vi "Read_Temp_Omega.vi"(11 "VISA Omega (Serial - COM1)":refnum<visa-resource-name>) -> (0 "error out":errorcluster, 3 "Temperature":dbl)   [LabVIEW 2012]
uses:
  <vilib>/Instr/_visa.llb/VISA Configure Serial Port (Instr).vi
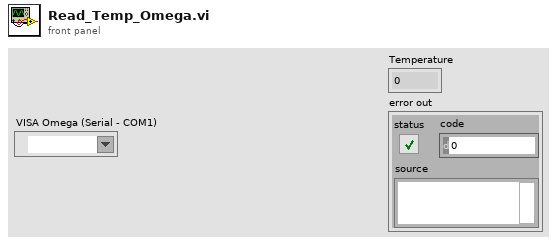
[diagram p1: front panel]
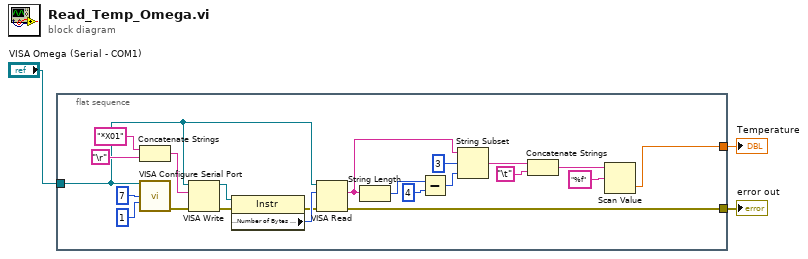
[diagram p0: block diagram]
diagram:
  n1 = flat-sequence {
    tunnel: "VISA Omega (Serial - COM1)" -> [w6]
    tunnel: [w5] -> w1
    tunnel: [w4] -> w2
    frame #0 {
      n2 = Concatenate Strings("*X01", "\r") -> (w14:string)
      n3 = call-poly "VISA Configure Serial Port"("VISA resource name"=w6, "data bits (8)"=7, "parity (0:none)"=1) -> ("error out"=w11:errorcluster)  [unwired: 11 in, 1 out]
      n4 = VISA Write(VISA resource name=w6, write buffer=w14, error in (no error)=w11) -> (VISA resource name out=w25:refnum<visa-resource-name>, error out=w15:errorcluster)  [unwired: 1 out]
      n5 = property class="Instr"(reference=w25, error in=w15) -> (error out=w16:errorcluster, "Serial Settings:Number of Bytes at Serial Port"=w17:u32)  [unwired: 1 out]
      n6 = VISA Read(VISA resource name=w6, byte count=w17, error in (no error)=w16) -> (read buffer=w18:string, error out=w5:errorcluster)  [unwired: 2 out]
      n7 = String Length(string=w18) -> (length=w20:i32)
      n8 = Subtract(x=w20, y=4) -> (x-y=w22:i32)
      n9 = String Subset(string=w18, offset (0)=3, length (rest)=w22) -> (substring=w23:string)
      n10 = Concatenate Strings(w23, "\t") -> (w7:string)
      n11 = Scan Value(string=w7, format string="%f") -> (value=w4:dbl)  [unwired: 1 in, 1 out]
    }
  }
  "Temperature" <- w2
  "error out" <- w1
